vi "add module to engine.vi"(8 "error in":errorcluster, 10 "module ID":string, 11 "Standard Engine Configuration in":refnum<class "Standard Engine Configuration.lvclass">) -> (0 "error out":errorcluster, 3 "Standard Engine Configuration out":refnum<class "Standard Engine Configuration.lvclass">)   [LabVIEW 2013, in "Standard Engine Configuration.lvclass"]
doc: "Adds a new module to the engine for it to execute."
uses:
  Standard Engine Configuration.lvclass
  Module Decimation.ctl
  <vilib>/NI/Module Execution Interface/Engine Configuration/engine configuration.lvclass
  Standard Engine Configuration.lvclass/Standard Engine Configuration.ctl
  Module Specific Configuration.ctl
  Runtime/error responses.ctl
  error options.ctl
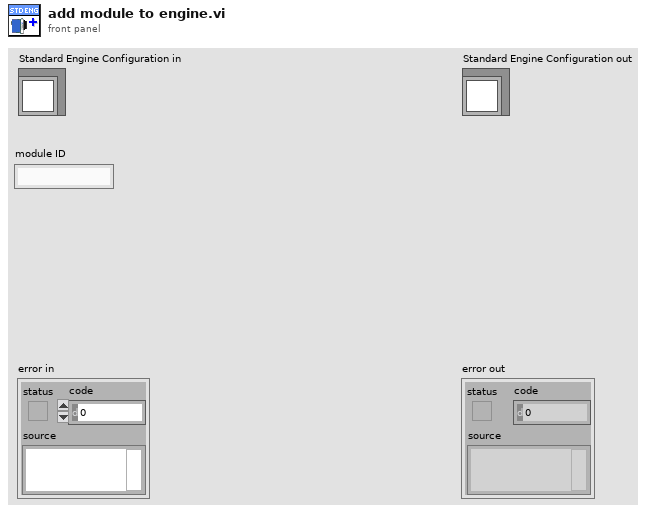
[diagram p1: front panel]
types:
  T1 = typedef "Standard Engine Configuration.lvclass/Module Decimation.ctl" = cluster{"Decimation":u16, "Offset":u16, "sort order":i32, "async?":bool}
  T2 = typedef "Standard Engine Configuration.lvclass/Module Specific Configuration.ctl" = cluster{"Module ID":string, "Module Decimation":T1, "error tag":string, "error responses":T3}
  T3 = typedef "Standard Engine Configuration.lvclass/error responses.ctl" = cluster{"unknown":T4, "trivial":T4, "critical":T4, "recoverable":T4}
  T4 = typedef "Standard Engine Configuration.lvclass/error options.ctl" = cluster{"clear":bool, "notify":bool, "log":bool, "remove module":bool, "abort engine":bool, "go to safe state":bool, "recover module":bool}
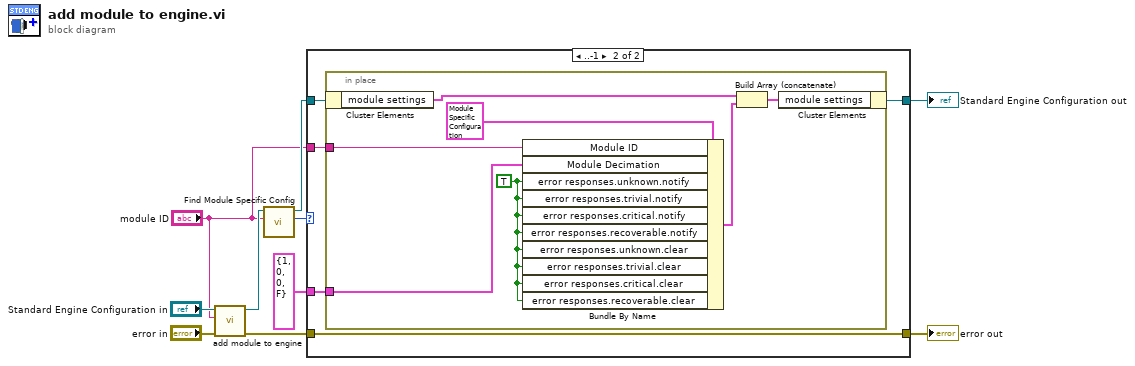
[diagram p0: block diagram]
diagram:
  n1 = call-parent "add module to engine.vi"("error in"="error in", "module ID"="module ID", "engine configuration in"="Standard Engine Configuration in") -> ("error out"=w4:errorcluster, "engine configuration out"=w2:refnum<class "Standard Engine Configuration.lvclass">)  [unwired: 7 in]
  n2 = call "Find Module Specific Config.vi"("Module ID"="module ID", "Standard Engine Repo Data in"=w2) -> ("Index"=w7:i32, "Standard Engine Repo Data out"=w9:refnum<class "Standard Engine Configuration.lvclass">)  [unwired: 8 in]
  n3 = case shown="..-1" w7 {
    tunnel: [w12 w17] -> w10
    tunnel: w9 -> [w12 w16]
    tunnel: w4 -> [w11 w15]
    tunnel: T1 {"Decimation"=1, "Offset"=0, "sort order"=0, "async?"=FALSE} ("module decimation") -> [_ w14]
    tunnel: [w11 w15] -> w5
    tunnel: "module ID" -> [_ w13]
    frame 0.. {
    }
    frame ..-1 {
      n4 = in-place {
        in-place-border: w14 -> [w20]
        in-place-border: w13 -> [w19]
        w18 = TRUE
        n5 = in-place-cluster #1(w16) -> ("module settings"=w23:T2[])
        n6 = Bundle By Name(cluster=T2 {"Module ID"="", "Module Decimation"={"Decimation"=0, "Offset"=0, "sort order"=0, "async?"=FALSE}, "error tag"="", "error responses"={"unknown"={"clear"=FALSE, "notify"=FALSE, "log"=FALSE, "remove module"=FALSE, "abort engine"=FALSE, "go to safe state"=FALSE, "recover module"=FALSE}, "trivial"={"clear"=FALSE, "notify"=FALSE, "log"=FALSE, "remove module"=FALSE, "abort engine"=FALSE, "go to safe state"=FALSE, "recover module"=FALSE}, "critical"={"clear"=FALSE, "notify"=FALSE, "log"=FALSE, "remove module"=FALSE, "abort engine"=FALSE, "go to safe state"=FALSE, "recover module"=FALSE}, "recoverable"={"clear"=FALSE, "notify"=FALSE, "log"=FALSE, "remove module"=FALSE, "abort engine"=FALSE, "go to safe state"=FALSE, "recover module"=FALSE}}} ("Module Specific Configuration"), "Module ID"=w19, "Module Decimation"=w20, "error responses.unknown.notify"=w18, "error responses.trivial.notify"=w18, "error responses.critical.notify"=w18, "error responses.recoverable.notify"=w18, "error responses.unknown.clear"=w18, "error responses.trivial.clear"=w18, "error responses.critical.clear"=w18, "error responses.recoverable.clear"=w18) -> (w21:T2)
        n7 = Build Array (concatenate)(w23, w21) -> (w22:T2[])
        n8 = in-place-cluster #1("module settings"=w22) -> (w17:refnum<class "Standard Engine Configuration.lvclass">)
      }
    }
  }
  "error out" <- w5
  "Standard Engine Configuration out" <- w10
